vi "Teleop.vi"(1 "PreValue 2":bool, 3 "PreValue":bool, 9 "PreValue 3":bool, 10 "Match Info":T1={"Autonomous Elapsed Seconds"=0.0, "TeleOp Elapsed Seconds"=0.0, "Disabled Elapsed Seconds"=0.0, "Visited Autonomous"=FALSE, "Visited TeleOp"=FALSE, "Visited Disabled"=FALSE, "Autonomous Settings"={"Autonomous Style"=enum."Independent", "VI Refnum"=refnum}}, 11 "Call Context":T2) -> (0 "CurrentValue 2":bool, 2 "CurrentValue":bool, 8 "CurrentValue 3":bool)   [LabVIEW 2015]
doc: "This VI is called for each TeleOp packet received from the DS where the robot is not disabled. It is often used to read from the joysticks and update I/O or to update setpoints for timed control loops. It should complete and return within 20 milliseconds or it may miss DS packets."
uses:
  <vilib>/Rock Robotics/WPI/DriverStation/WPI_DriverStationDerivedRobotMode.ctl
  <vilib>/Rock Robotics/WPI/DriverStation/WPI_DriverStationMatch Info.ctl
  <vilib>/Rock Robotics/WPI/Solenoid/WPI_SolenoidValue.ctl
  <vilib>/Rock Robotics/WPI/Utilities/WPI_GetSetVariantRefNum.vi
  <vilib>/Rock Robotics/Network Tables/NT Write Boolean.vi
  <vilib>/Rock Robotics/Network Tables/NT Write Numeric Array.vi
  <vilib>/Rock Robotics/Network Tables/NT Read Boolean.vi
  <vilib>/Rock Robotics/Network Tables/NT Read Number.vi
  <vilib>/Rock Robotics/WPI/Solenoid/WPI_SolenoidSetEnum.vi
panel:
  out "Sample Slider 0":dbl(slide) scale=0.0..5.0
  out "Sample Boolean 1":bool
  out "Sample Boolean 0":bool
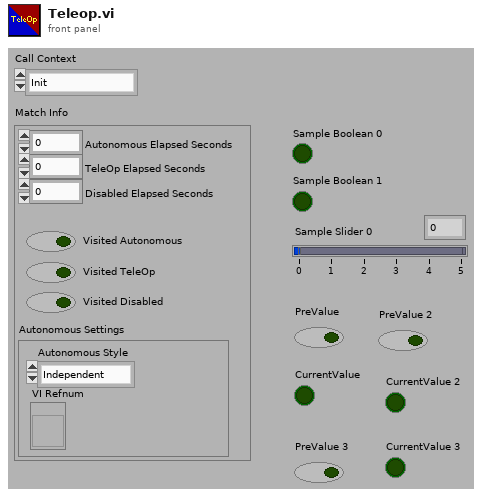
[diagram p1: front panel]
types:
  T1 = typedef "WPI_DriverStationMatch Info.ctl" = cluster{"Autonomous Elapsed Seconds":dbl, "TeleOp Elapsed Seconds":dbl, "Disabled Elapsed Seconds":dbl, "Visited Autonomous":bool, "Visited TeleOp":bool, "Visited Disabled":bool, "Autonomous Settings":cluster{"Autonomous Style":enum16{"Iterative", "Independent"}, "VI Refnum":refnum<vi>}}
  T2 = typedef "WPI_DriverStationDerivedRobotMode.ctl" = enum16{"Init", "Execute", "Stop"}
  T3 = typedef "WPI_SolenoidValue.ctl" = enum16{"Off", "On", "Forward", "Reverse"}
  T4 = typedef "WPI_JoystickDevRef.ctl" = cluster{"Device":T5}
  T5 = typedef "WPI_JoystickDeviceEnum.ctl" = enum16{"USB 0", "USB 1", "USB 2", "USB 3", "USB 4", "USB 5"}
  T6 = cluster{"Buttons[0]":bool, "Buttons[1]":bool, "Buttons[2]":bool, "Buttons[3]":bool, "Buttons[4]":bool, "Buttons[5]":bool, "Buttons[6]":bool, "Buttons[7]":bool, "Buttons[8]":bool}
  T7 = typedef "WPI_RobotDriveDevRef.ctl" = cluster{"DevStatus":errorcluster, "Motors[]":T8[], "Square Inputs":bool, "Max Output":dbl}
  T8 = typedef "WPI_MotorControlDeviceRef.ctl" = cluster{"DeviceStatus":errorcluster, "Type":T9, "PWM":cluster{"PWM Channel":T10, "DeadBand":T11}, "CAN":cluster{"Device Number":u8, "Control Mode":T12, "Semaphore":T13, "Max Vout":dbl, "TalonSRX Control Mode":T14}, "Invert":bool}
  T9 = typedef "WPI_MotorControlType.ctl" = enum16{"PWM", "CAN", "CANTalonSRX"}
  T10 = typedef "FPGA_DIOPWMChannel.ctl" = enum8{"PWM 0", "PWM 1", "PWM 2", "PWM 3", "PWM 4", "PWM 5", "PWM 6", "PWM 7", "PWM 8", "PWM 9", "PWM MXP 0", "PWM MXP 1", "PWM MXP 2", "PWM MXP 3", "PWM MXP 4", "PWM MXP 5", "PWM MXP 6", "PWM MXP 7", "PWM MXP 8", "PWM MXP 9", "Invalid"}
  T11 = typedef "WPI_PWMDeadband.ctl" = cluster{"Name":string, "maxPositivePwm":i32, "minPositivePwm":i32, "centerPwm":i32, "maxNegativePwm":i32, "minNegativePwm":i32, "angularRange":u16}
  T12 = typedef "WPI_CANJaguar_ControlMode.ctl" = enum8{"Percent VBus", "Current", "Speed", "Position", "Voltage"}
  T13 = typedef "Semaphore RefNum" = refnum<k1>
  T14 = typedef "WPI_CANTalonSRX_APIControlMode.ctl" = enum8{"Percent VBus", "Speed", "Position", "Slave", "Unchanged / Invalid", "Voltage Compensation", "Current", "Motion Profile"}
  T15 = typedef "WPI_SolenoidDevRef.ctl" = cluster{"DevStatus":errorcluster, "Pneumatics Control Module":u8, "Forward Solenoid Channel":T16, "Reverse Solenoid Channel":T16}
  T16 = typedef "WPI_SolenoidChannel.ctl" = enum8{"Solenoid 0", "Solenoid 1", "Solenoid 2", "Solenoid 3", "Solenoid 4", "Solenoid 5", "Solenoid 6", "Solenoid 7", "Invalid"}
  T17 = typedef "WPI_DigitalInputDevRef.ctl" = cluster{"DevStatus":errorcluster, "DIO Channel":T18}
  T18 = typedef "FPGA_DIOChannel.ctl" = enum8{"DIO 0", "DIO 1", "DIO 2", "DIO 3", "DIO 4", "DIO 5", "DIO 6", "DIO 7", "DIO 8", "DIO 9", "DIO MXP 0", "DIO MXP 1", "DIO MXP 2", "DIO MXP 3", "DIO MXP 4", "DIO MXP 5", "DIO MXP 6", "DIO MXP 7", "DIO MXP 8", "DIO MXP 9", "DIO MXP 10", "DIO MXP 11", "DIO MXP 12", "DIO MXP 13", "DIO MXP 14", "DIO MXP 15", "Invalid"}
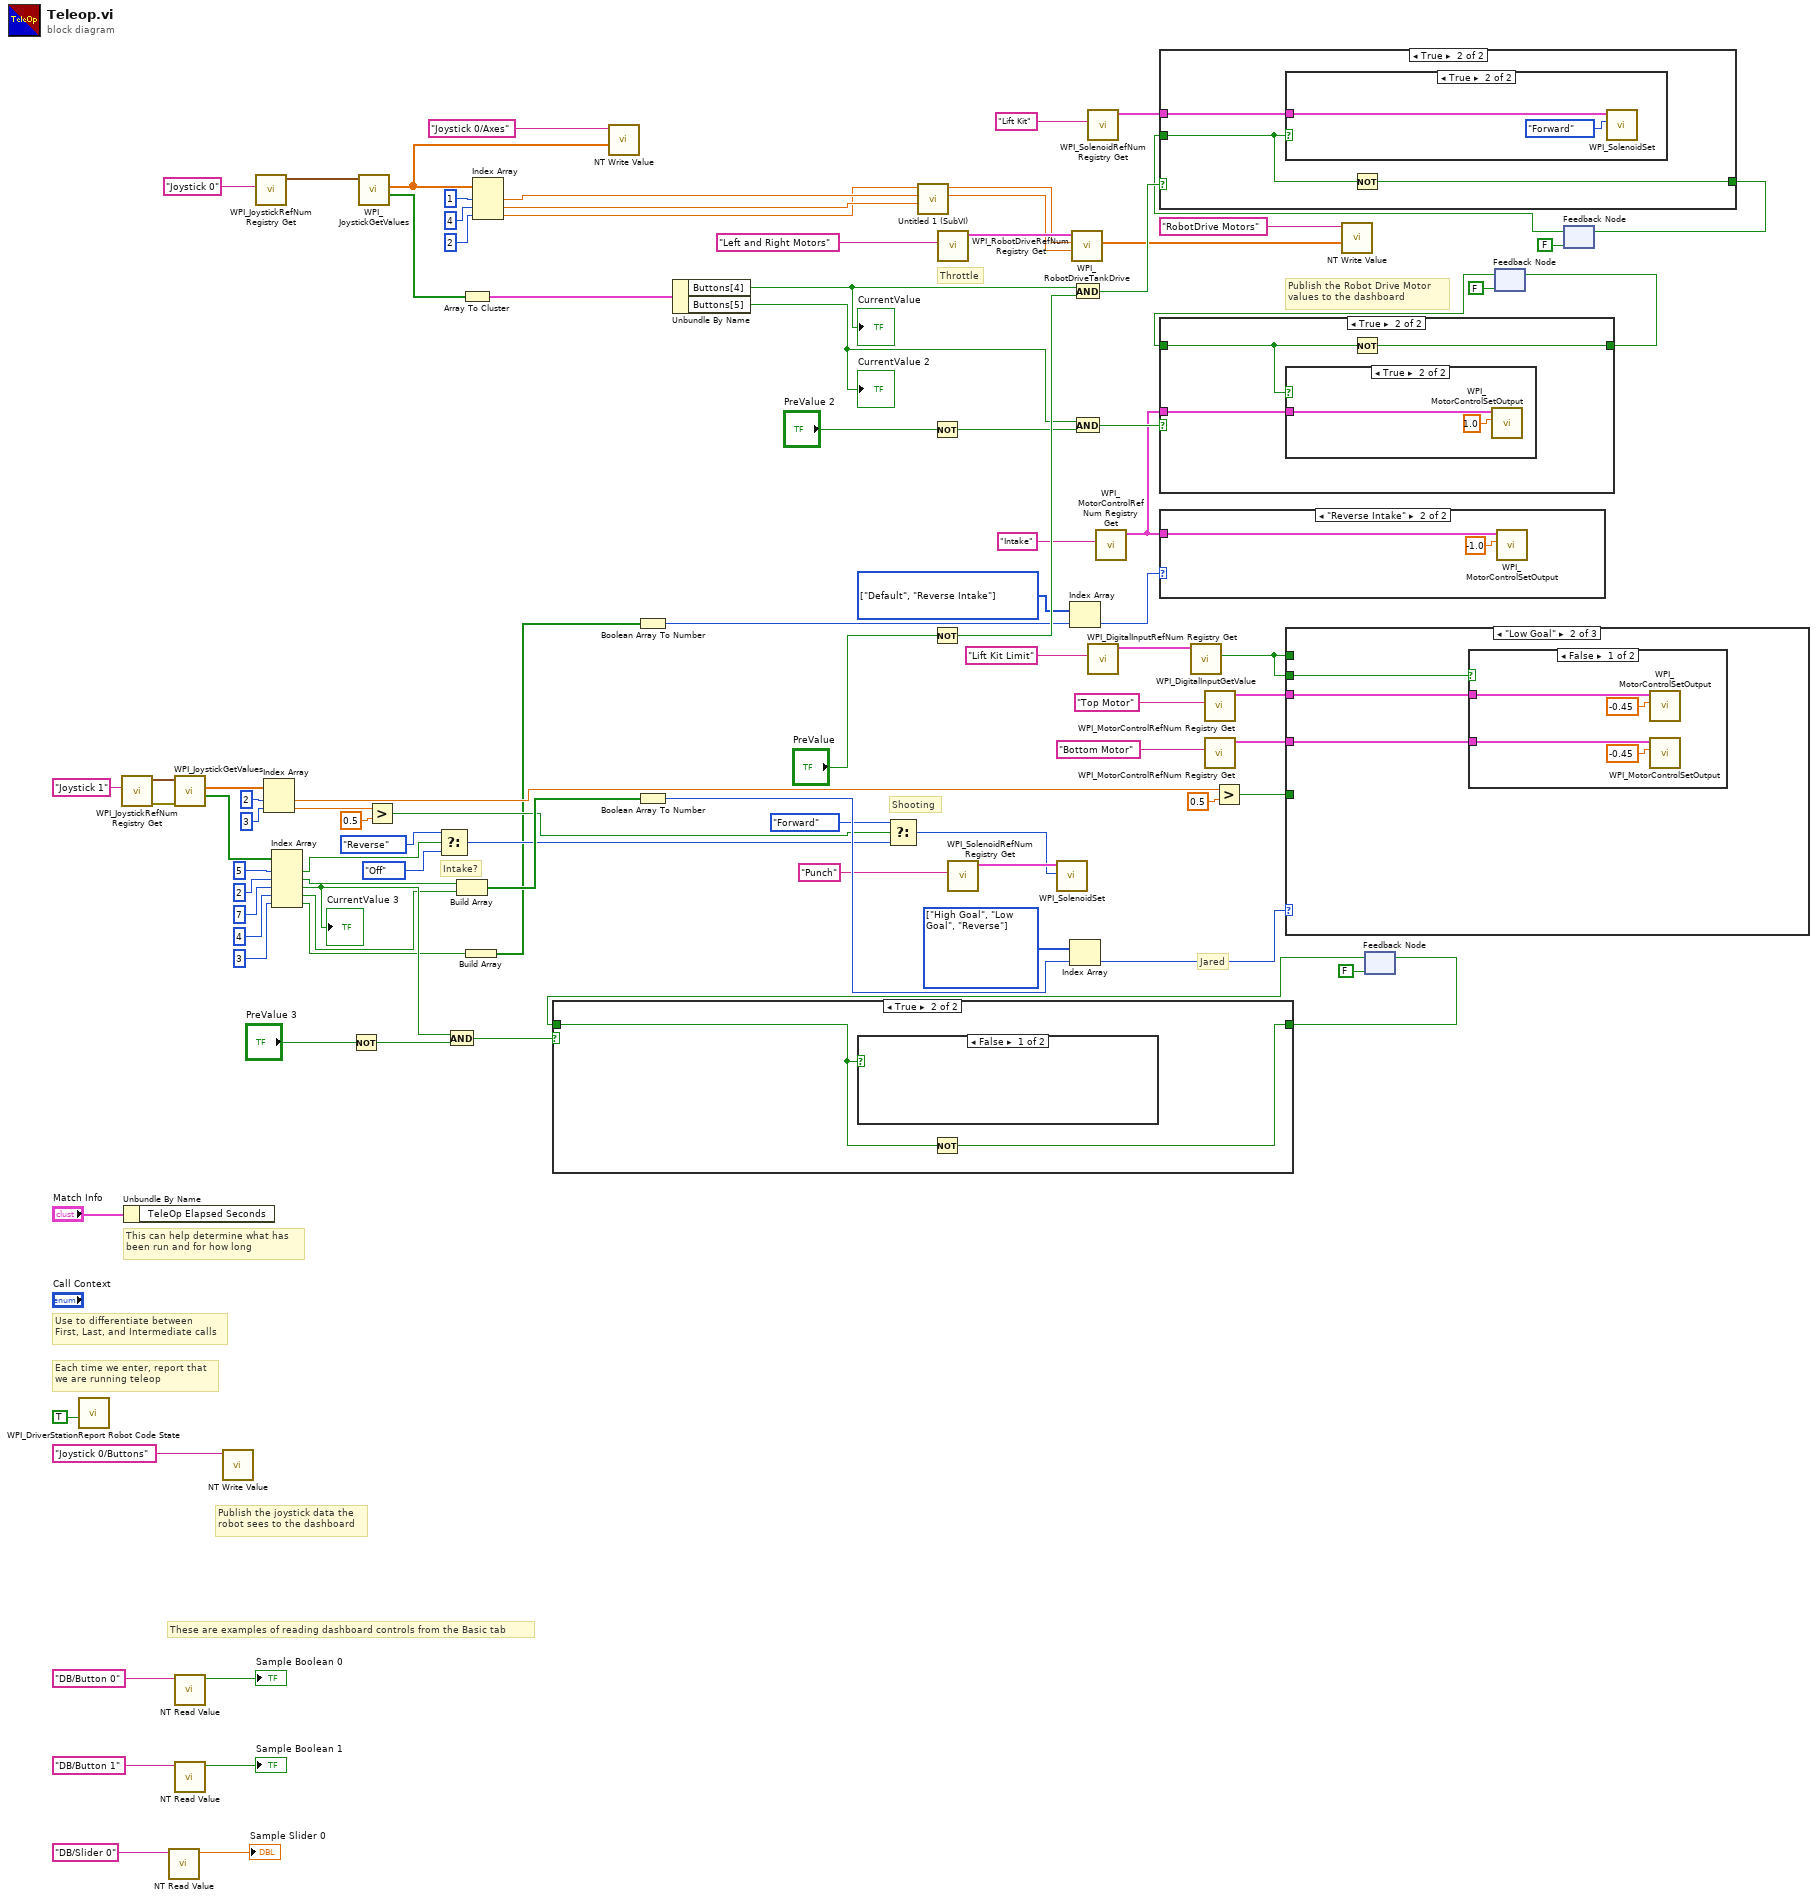
[diagram p0: block diagram]
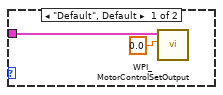
[diagram p2: hidden frame]
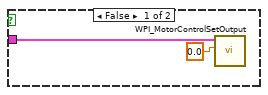
[diagram p6: hidden frame]
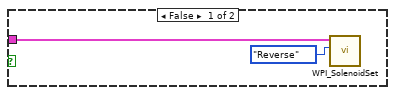
[diagram p8: hidden frame]
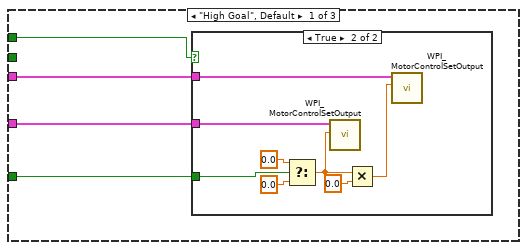
[diagram p9: hidden frame]
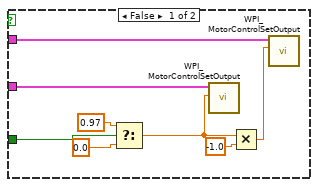
[diagram p10: hidden frame]
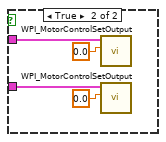
[diagram p11: hidden frame]
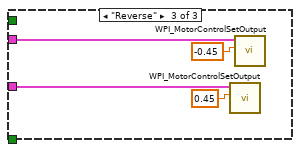
[diagram p12: hidden frame]
diagram:
  w2 = enum16{"Default", "Reverse Intake"}[] [enum."Default", enum."Reverse Intake"] items=["Default", "Reverse Intake"] ("array")
  w78 = enum16{"High Goal", "Low Goal", "Reverse", ""}[] [enum."High Goal", enum."Low Goal", enum."Reverse"] items=["High Goal", "Low Goal", "Reverse", ""] ("array")
  # "Jared"
  # "Intake?"
  # "Shooting"
  # "Throttle"
  # "These are examples of reading dashboard controls from the Basic tab"
  # "Publish the Robot Drive Motor\nvalues to the dashboard"
  # "Publish the joystick data the\nrobot sees to the dashboard"
  # "Each time we enter, report that\nwe are running teleop"
  # "Use to differentiate between\nFirst, Last, and Intermediate calls"
  # "This can help determine what has\nbeen run and for how long"
  n1 = call <vilib>:"WPI_DriverStationReport Robot Code State.vi"("TeleOp"=TRUE ("Autonomous")) -> ()  [unwired: 10 in, 1 out]
  n2 = call <vilib>:"WPI_JoystickRefNum Registry Get.vi"("refnum name"="Joystick 1") -> ("error out"=w55:errorcluster, "JoystickDevRef"=w54:T4)  [unwired: 1 in, 8 out]
  n3 = Unbundle By Name("Match Info") -> ()  [unwired: 1 out]
  n4 = call-poly <vilib>:"NT Read Value.vi"("Name"="DB/Slider 0" ("refnum name")) -> ("Numeric"=→"Sample Slider 0":dbl)  [unwired: 9 in, 1 out]
  n5 = call <vilib>:"WPI_JoystickGetValues.vi"("error in (no error)"=w55, "JoystickDevRef"=w54) -> ("Buttons"=w17:bool[], "Axes"=w52:dbl[])  [unwired: 5 in, 3 out]
  n6 = call-poly <vilib>:"NT Read Value.vi"("Name"="DB/Button 0" ("refnum name")) -> ("Boolean"=→"Sample Boolean 0":bool)  [unwired: 9 in, 1 out]
  n7 = call-poly <vilib>:"NT Read Value.vi"("Name"="DB/Button 1" ("refnum name")) -> ("Boolean"=→"Sample Boolean 1":bool)  [unwired: 9 in, 1 out]
  n8 = call-poly <vilib>:"NT Write Value.vi"("Name"="Joystick 0/Buttons") -> ()  [unwired: 10 in, 1 out]
  n9 = call <vilib>:"WPI_JoystickRefNum Registry Get.vi"("refnum name"="Joystick 0") -> ("JoystickDevRef"=w93:T4)  [unwired: 1 in, 9 out]
  n10 = Index Array(array=w52, index #1=2 ("index"), index #2=3 ("index")) -> (element #1=w51:dbl, element #2=w46:dbl)
  n11 = Index Array(array=w17, index #1=5 ("index"), index #2=2 ("index"), index #3=7 ("index"), index #4=4 ("index"), index #5=3 ("index")) -> (element #1=w9:bool, element #2=w23:bool, element #3=w29:bool, element #4=w21:bool, element #5=w4:bool)
  "CurrentValue 3" <- w29
  n12 = Not(x="PreValue 3") -> (.not. x?=w30:bool)
  n13 = call <vilib>:"WPI_JoystickGetValues.vi"("JoystickDevRef"=w93) -> ("Buttons"=w74:bool[], "Axes"=w89:dbl[])  [unwired: 6 in, 3 out]
  n14 = Greater?(x=w46, y=0.5) -> (0:w8:bool)
  n15 = Select(t=WPI_SolenoidValue."Reverse" ("Value"), s=w9, f=WPI_SolenoidValue."Off" ("Value")) -> (s? t:f=w12:T3)
  n16 = And(x=w29, y=w30) -> (x .and. y?=w28:bool)
  n17 = Build Array(w23, w21) -> (w80:bool[])
  n18 = Array To Cluster(array=w74) -> (cluster=w81:T6)
  n19 = Build Array(w4) -> (w3:bool[])
  n20 = Index Array(array=w89, index #1=1 ("index"), index #2=4 ("index"), index #3=2 ("index")) -> (element #1=w36:dbl, element #2=w37:dbl, element #3=w35:dbl)
  n21 = call-poly <vilib>:"NT Write Value.vi"("Numeric Array"=w89, "Name"="Joystick 0/Axes") -> ()  [unwired: 9 in, 1 out]
  n22 = Boolean Array To Number(Boolean array=w3) -> (number=w6:u32)
  n23 = Boolean Array To Number(Boolean array=w80) -> (number=w79:u32)
  n24 = Unbundle By Name(w81) -> ("Buttons[4]"=w71:bool, "Buttons[5]"=w40:bool)
  "CurrentValue" <- w71
  "CurrentValue 2" <- w40
  n25 = Select(t=WPI_SolenoidValue."Forward" ("Value"), s=w8, f=w12) -> (s? t:f=w15:T3)
  n26 = call "Untitled 1 (SubVI).vi"("upper limit 2"=w37, "upper limit"=w36, "Throttle"=w35) -> ("Numeric 2"=w60:dbl, "Numeric"=w59:dbl)  [unwired: 7 in]
  n27 = Not(x="PreValue 2") -> (.not. x?=w39:bool)
  n28 = Not(x="PreValue") -> (.not. x?=w69:bool)
  n29 = call <vilib>:"WPI_RobotDriveRefNum Registry Get.vi"("refnum name"="Left and Right Motors") -> ("RobotDriveDevRef"=w61:T7)  [unwired: 1 in, 9 out]
  n30 = call <vilib>:"WPI_SolenoidRefNum Registry Get.vi"("refnum name"="Punch") -> ("SolenoidDevRef"=w16:T15)  [unwired: 9 in, 1 out]
  n31 = call-poly <vilib>:"WPI_SolenoidSet.vi"("Value"=w15, "SolenoidDevRef"=w16) -> ()  [unwired: 8 in, 2 out]
  n32 = Index Array(array=w2, index=w6) -> (element=w1:enum16{"Default", "Reverse Intake"})
  n33 = Index Array(array=w78, index=w79) -> (element=w77:enum16{"High Goal", "Low Goal", "Reverse", ""})
  n34 = call <vilib>:"WPI_RobotDriveTankDrive.vi"("Right axis value"=w60, "Left axis value"=w59, "RobotDriveDevRef"=w61) -> ("Motor Values"=w62:dbl[])  [unwired: 6 in, 2 out]
  n35 = And(x=w71, y=w69) -> (x .and. y?=w68:bool)
  n36 = And(x=w40, y=w39) -> (x .and. y?=w38:bool)
  n37 = call <vilib>:"WPI_SolenoidRefNum Registry Get.vi"("refnum name"="Lift Kit") -> ("SolenoidDevRef"=w63:T15)  [unwired: 9 in, 1 out]
  n38 = call <vilib>:"WPI_DigitalInputRefNum Registry Get.vi"("refnum name"="Lift Kit Limit") -> ("DigitalInputDevRef"=w20:T17)  [unwired: 9 in, 1 out]
  n39 = call <vilib>:"WPI_MotorControlRefNum Registry Get.vi"("refnum name"="Intake") -> ("MotorControlDevRef"=w7:T8)  [unwired: 9 in, 1 out]
  n40 = case shown="\"Reverse Intake\"" w1 {
    tunnel: w7 -> [w98 w100]
    frame "Default", Default {
      n41 = call <vilib>:"WPI_MotorControlSetOutput.vi"("Output"=0.0, "MotorControlDevRef"=w98) -> ()  [unwired: 7 in, 3 out]
    }
    frame "Reverse Intake" {
      n42 = call <vilib>:"WPI_MotorControlSetOutput.vi"("Output"=-1.0, "MotorControlDevRef"=w100) -> ()  [unwired: 7 in, 3 out]
    }
  }
  n43 = call <vilib>:"WPI_DigitalInputGetValue.vi"("DigitalInputDevRef"=w20) -> ("Value"=w18:bool)  [unwired: 8 in, 2 out]
  n44 = call <vilib>:"WPI_MotorControlRefNum Registry Get.vi"("refnum name"="Top Motor") -> ("MotorControlDevRef"=w72:T8)  [unwired: 9 in, 1 out]
  n45 = call <vilib>:"WPI_MotorControlRefNum Registry Get.vi"("refnum name"="Bottom Motor") -> ("MotorControlDevRef"=w76:T8)  [unwired: 9 in, 1 out]
  n46 = Greater?(x=w51, y=0.5) -> (0:w49:bool)
  n47 = case shown="\"Low Goal\"" w77 {
    tunnel: w76 -> [w104 w123 w134]
    tunnel: w72 -> [w103 w122 w132]
    tunnel: w49 -> [w102 _ _]
    tunnel: w18 -> [_ w121 _]
    tunnel: w18 -> [w101 _ _]
    frame "High Goal", Default {
      n48 = case shown="True" w101 {
        tunnel: w104 -> [w106 w120]
        tunnel: w103 -> [w105 w119]
        tunnel: w102 -> [w111 w118]
        frame False {
          n49 = Select(t=0.97, s=w111, f=0.0) -> (s? t:f=w110:dbl)
          n50 = call <vilib>:"WPI_MotorControlSetOutput.vi"("Output"=w110, "MotorControlDevRef"=w106) -> ()  [unwired: 7 in, 3 out]
          n51 = Multiply(x=w110, y=-1.0) -> (x*y=w112:dbl)
          n52 = call <vilib>:"WPI_MotorControlSetOutput.vi"("Output"=w112, "MotorControlDevRef"=w105) -> ()  [unwired: 7 in, 3 out]
        }
        frame True {
          n53 = Select(t=0.0, s=w118, f=0.0) -> (s? t:f=w116:dbl)
          n54 = call <vilib>:"WPI_MotorControlSetOutput.vi"("Output"=w116, "MotorControlDevRef"=w120) -> ()  [unwired: 7 in, 3 out]
          n55 = Multiply(x=w116, y=0.0) -> (x*y=w114:dbl)
          n56 = call <vilib>:"WPI_MotorControlSetOutput.vi"("Output"=w114, "MotorControlDevRef"=w119) -> ()  [unwired: 7 in, 3 out]
        }
      }
    }
    frame "Low Goal" {
      n57 = case shown="False" w121 {
        tunnel: w123 -> [w124 w130]
        tunnel: w122 -> [w125 w128]
        frame False {
          n58 = call <vilib>:"WPI_MotorControlSetOutput.vi"("Output"=-0.45, "MotorControlDevRef"=w125) -> ()  [unwired: 7 in, 3 out]
          n59 = call <vilib>:"WPI_MotorControlSetOutput.vi"("Output"=-0.45, "MotorControlDevRef"=w124) -> ()  [unwired: 7 in, 3 out]
        }
        frame True {
          n60 = call <vilib>:"WPI_MotorControlSetOutput.vi"("Output"=0.0, "MotorControlDevRef"=w128) -> ()  [unwired: 7 in, 3 out]
          n61 = call <vilib>:"WPI_MotorControlSetOutput.vi"("Output"=0.0, "MotorControlDevRef"=w130) -> ()  [unwired: 7 in, 3 out]
        }
      }
    }
    frame "Reverse" {
      n62 = call <vilib>:"WPI_MotorControlSetOutput.vi"("Output"=0.45, "MotorControlDevRef"=w134) -> ()  [unwired: 7 in, 3 out]
      n63 = call <vilib>:"WPI_MotorControlSetOutput.vi"("Output"=-0.45, "MotorControlDevRef"=w132) -> ()  [unwired: 7 in, 3 out]
    }
  }
  n64 = call-poly <vilib>:"NT Write Value.vi"("Numeric Array"=w62, "Name"="RobotDrive Motors") -> ()  [unwired: 9 in, 1 out]
  n65 = feedback #1(FALSE) -> (w25:bool)
  n66 = case shown="True" w28 {
    tunnel: [w136 w138] -> w26
    tunnel: w25 -> [w136 w137]
    frame False {
    }
    frame True {
      n67 = case shown="False" w137 {
        frame False {
        }
        frame True {
        }
      }
      n68 = Not(x=w137) -> (.not. x?=w138:bool)
    }
  }
  n69 = feedback-in #1(w26) -> ()
  n70 = feedback #2(FALSE) -> (w42:bool)
  n71 = case shown="True" w38 {
    tunnel: [w139 w142] -> w43
    tunnel: w42 -> [w139 w140]
    tunnel: w7 -> [_ w141]
    frame False {
    }
    frame True {
      n72 = case shown="True" w140 {
        tunnel: w141 -> [w144 w146]
        frame False {
          n73 = call <vilib>:"WPI_MotorControlSetOutput.vi"("Output"=0.0, "MotorControlDevRef"=w144) -> ()  [unwired: 7 in, 3 out]
        }
        frame True {
          n74 = call <vilib>:"WPI_MotorControlSetOutput.vi"("Output"=1.0, "MotorControlDevRef"=w146) -> ()  [unwired: 7 in, 3 out]
        }
      }
      n75 = Not(x=w140) -> (.not. x?=w142:bool)
    }
  }
  n76 = feedback-in #2(w43) -> ()
  n77 = feedback #3(FALSE) -> (w65:bool)
  n78 = case shown="True" w68 {
    tunnel: [w147 w150] -> w66
    tunnel: w65 -> [w147 w148]
    tunnel: w63 -> [_ w149]
    frame False {
    }
    frame True {
      n79 = case shown="True" w148 {
        tunnel: w149 -> [w152 w154]
        frame False {
          n80 = call-poly <vilib>:"WPI_SolenoidSet.vi"("Value"=WPI_SolenoidValue."Reverse", "SolenoidDevRef"=w152) -> ()  [unwired: 8 in, 2 out]
        }
        frame True {
          n81 = call-poly <vilib>:"WPI_SolenoidSet.vi"("Value"=WPI_SolenoidValue."Forward", "SolenoidDevRef"=w154) -> ()  [unwired: 8 in, 2 out]
        }
      }
      n82 = Not(x=w148) -> (.not. x?=w150:bool)
    }
  }
  n83 = feedback-in #3(w66) -> ()
